vi "Check Is Helper Already Running (Get Queue) -- Wrapper.vi"(7 "Create? (F: Check)":bool, 8 "error in (no error)":errorcluster, 11 "JKI SM in":refnum<class "JKI SM.lvclass">) -> (0 "error out":errorcluster, 2 "is Running?":bool)   [LabVIEW 2013]
uses:
  JKI State Machine API/source/JKI SM/JKI SM.lvclass
  JKI State Machine API/source/JKI SM/JKI SM.lvclass/JKI SM.ctl
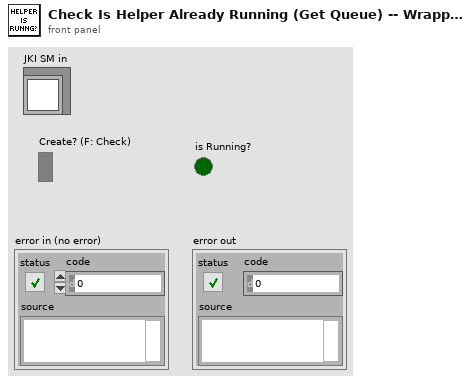
[diagram p1: front panel]
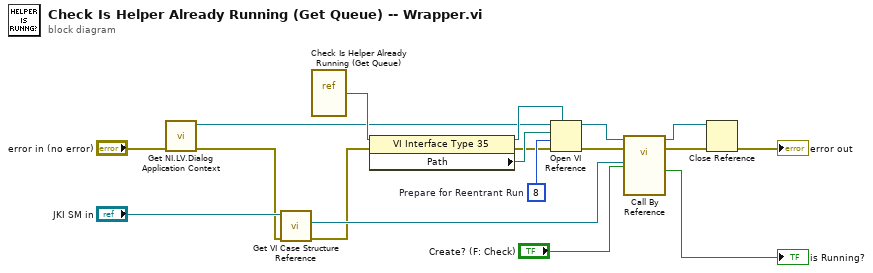
[diagram p0: block diagram]
diagram:
  w17 = 8  # Prepare for Reentrant Run
  n1 = call "Get NI.LV.Dialog Application Context.vi"("error in (no error)"="error in (no error)") -> ("error out"=w2:errorcluster, "Application out"=w5:refnum<vi>)  [unwired: 9 in]
  n2 = call "Get VI Case Structure Reference.vi"("error in (no error)"=w2, "JKI SM in"="JKI SM in") -> ("error out"=w1:errorcluster, "Case Structure ref"=w4:refnum<vi>)  [unwired: 7 in, 1 out]
  n3 = vi-ref "Check Is Helper Already Running (Get Queue).vi"() -> (w18:refnum<vi>)
  n4 = property class="VI Interface Type 35"(reference=w18, error in=w1) -> (reference out=w13:refnum<vi>, error out=w7:errorcluster, "Path"=w16:path)
  n5 = Open VI Reference(type specifier VI Refnum (for type only)=w13, application reference (local)=w5, vi path=w16, options=w17, error in (no error)=w7) -> (vi reference=w15:refnum<vi>, error out=w14:errorcluster)  [unwired: 1 out]
  n6 = call-by-ref "?"(reference=w15, error in=w14, "Create? (F: Check)"="Create? (F: Check)", "GObject in"=w4) -> (reference out=w11:refnum<vi>, error out=w12:errorcluster, "is Running?"=→"is Running?":bool)  [unwired: 9 in]
  n7 = Close Reference(reference=w11, error in (no error)=w12) -> (error out=→"error out":errorcluster)
